vi "pulse_generator_data.vi"(4 "Record dP Data":refnum<vi>, 5 "queue in":refnum<queue>, 6 "Stop! Refnum":refnum<vi>, 7 "Recording Progressbar":refnum<vi>, 8 "Seesion Start Time":timestamp, 9 "Pulse Generator Chart Refnums":T3, 10 "Pulse Generator Offsets and Data Saving Controls Refnums":T2, 11 "Pulse Generator Measurement Refnums":T1) -> ()   [LabVIEW 2015]
uses:
  <vilib>/DAQmx/configure/timing.llb/DAQmx Timing (Sample Clock).vi
  <vilib>/DAQmx/read.llb/DAQmx Read (Analog 1D Wfm NChan NSamp).vi
  <vilib>/Waveform/WDTOps.llb/WDT Get Waveform Time Array DBL.vi
  pulse_generator_data_controls_refnums.ctl
  pulse_generator_data_refnums.ctl
  pulse_generator_data_charts_refnums.ctl
panel:
  out "size(s)":i32[](graph)
  out "Sampling Rate":refnum<vi>
  out "Recording Duration":refnum<vi>
  out "Camera Voltage Chart":refnum<vi>
  out "Abs Tank Pressure Chart":refnum<vi>
  out "Pitot dP Chart":refnum<vi>
  out "Pulse Generator to Test Section dP Chart":refnum<vi>
  out "W1-7 dP":refnum<vi>
  out "W1-4 dP":refnum<vi>
  out "Mass Flow Rate":refnum<vi>
  out "Liquid Sat Pressure":refnum<vi>
  out "Liquid Temperature":refnum<vi>
  out "Vapor Sat Pressure":refnum<vi>
  out "Vapor Temperature":refnum<vi>
  out "Pitot dP":refnum<vi>
  out "PG to TS dP":refnum<vi>
  out "Pitot Current":refnum<vi>
  out "PG Abs Pressure":refnum<vi>
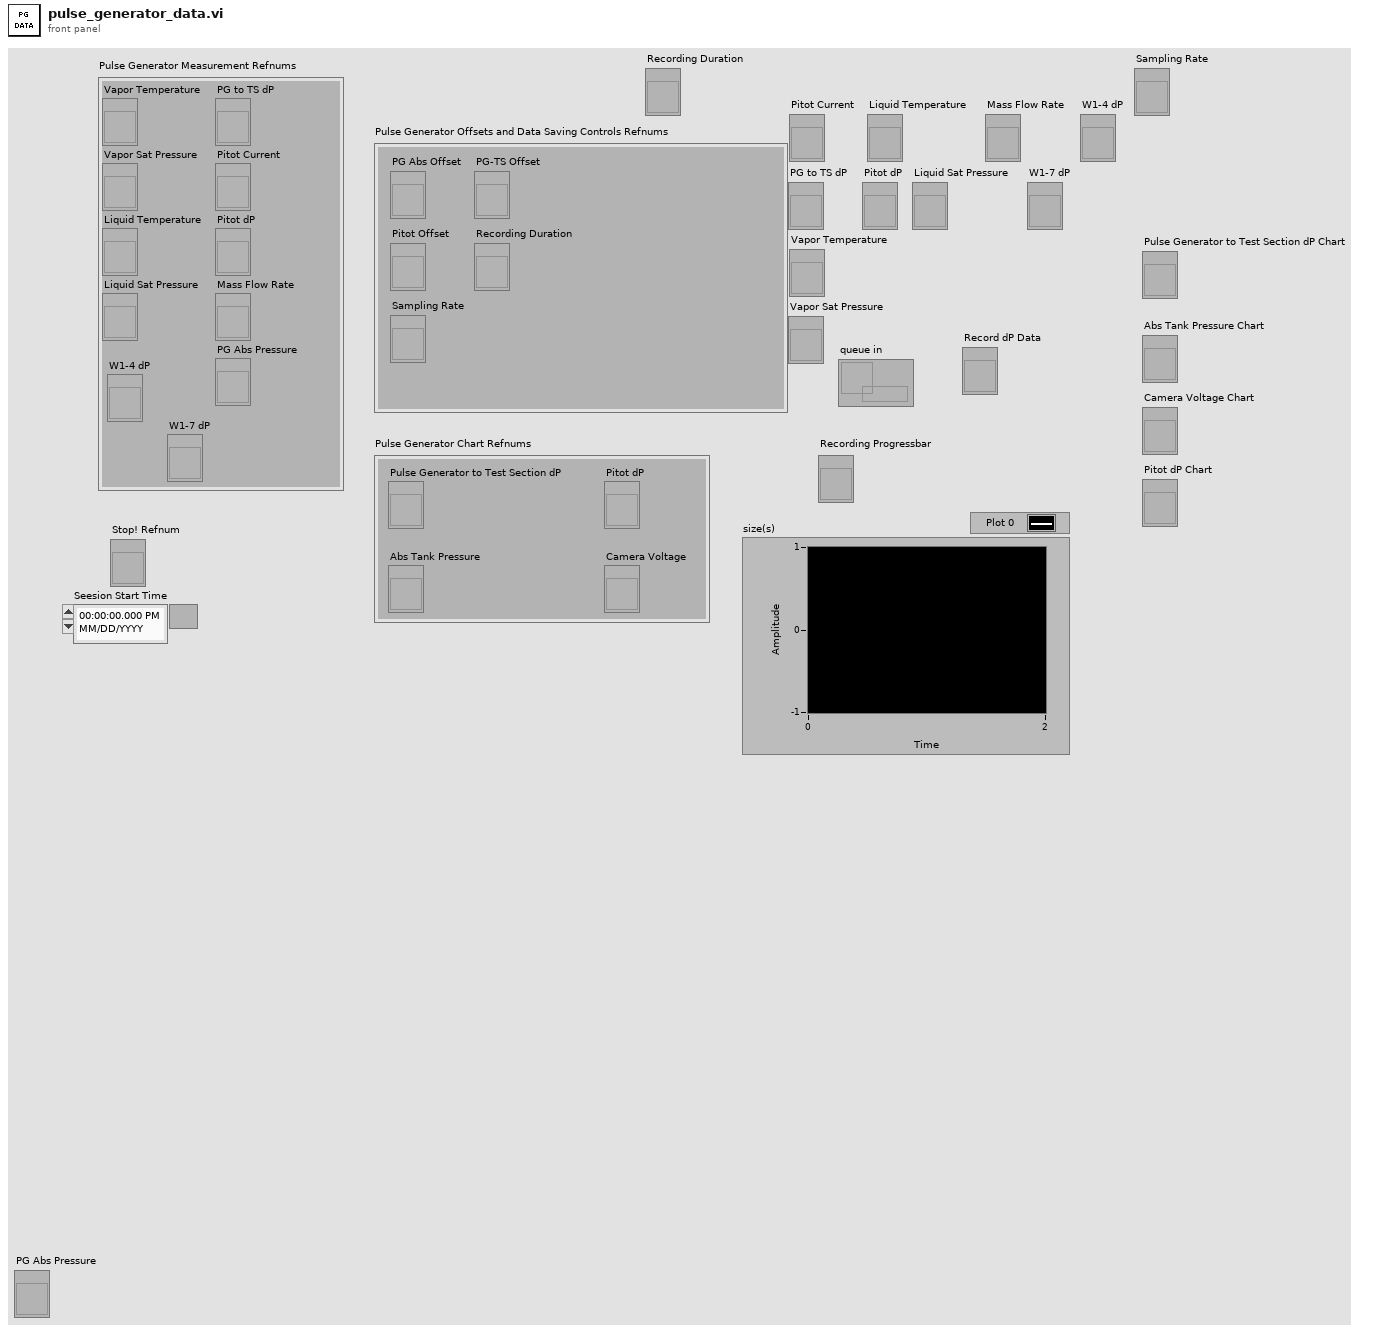
[diagram p1: front panel]
types:
  T1 = typedef "pulse_generator_data_refnums.ctl" = cluster{"Vapor Temperature":refnum<vi>, "Vapor Sat Pressure":refnum<vi>, "Liquid Temperature":refnum<vi>, "Liquid Sat Pressure":refnum<vi>, "PG to TS dP":refnum<vi>, "Pitot Current":refnum<vi>, "Pitot dP":refnum<vi>, "Mass Flow Rate":refnum<vi>, "PG Abs Pressure":refnum<vi>, "W1-4 dP":refnum<vi>, "W1-7 dP":refnum<vi>}
  T2 = typedef "pulse_generator_data_controls_refnums.ctl" = cluster{"PG Abs Offset":refnum<vi>, "Pitot Offset":refnum<vi>, "PG-TS Offset":refnum<vi>, "Recording Duration":refnum<vi>, "Sampling Rate":refnum<vi>}
  T3 = typedef "pulse_generator_data_charts_refnums.ctl" = cluster{"Pulse Generator to Test Section dP":refnum<vi>, "Pitot dP":refnum<vi>, "Abs Tank Pressure":refnum<vi>, "Camera Voltage":refnum<vi>}
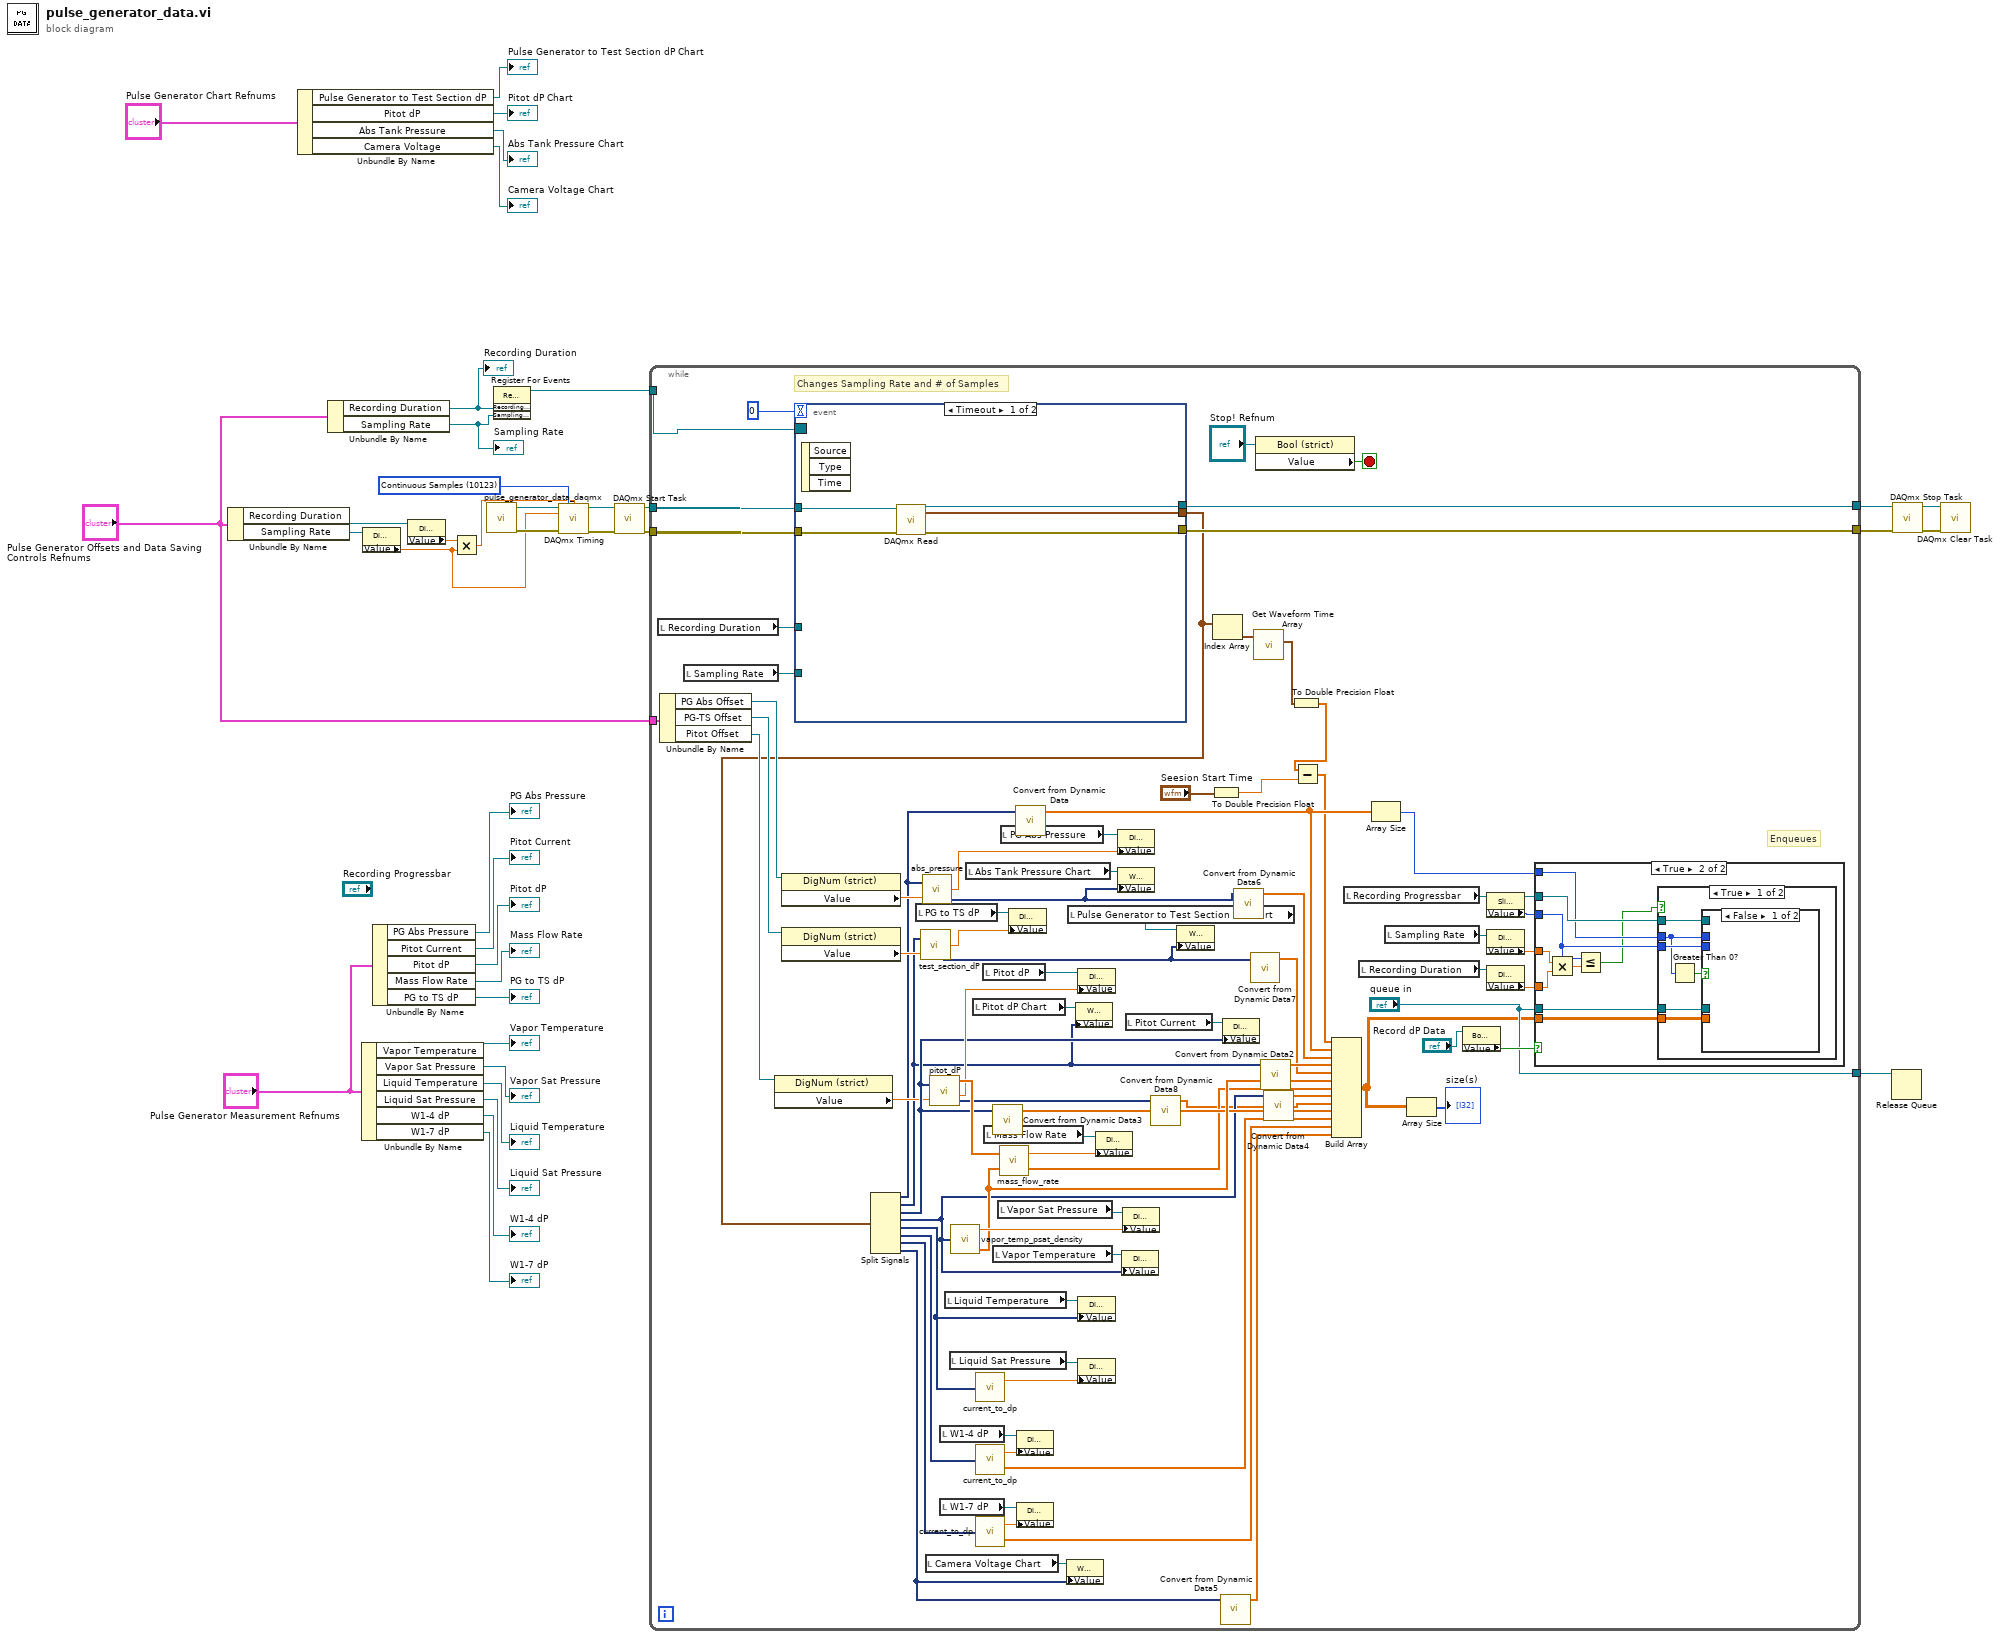
[diagram p0: block diagram]
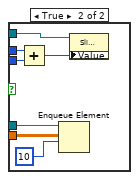
[diagram p3: hidden frame]
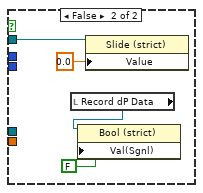
[diagram p4: hidden frame]
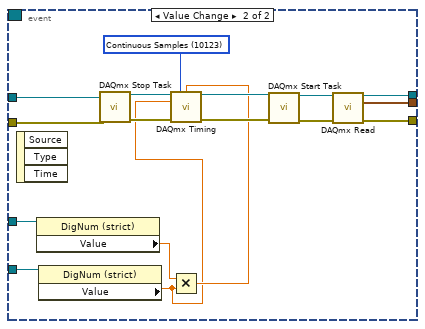
[diagram p5: hidden frame]
diagram:
  w34 = 10123 items=["Finite Samples"=10178, "Continuous Samples"=10123, "Hardware Timed Single Point"=12522] ("sample mode")
  n1 = Unbundle By Name("Pulse Generator Offsets and Data Saving Controls Refnums") -> ("Recording Duration"=w7:refnum<vi>, "Sampling Rate"=w2:refnum<vi>)
  n2 = Unbundle By Name("Pulse Generator Chart Refnums") -> ("Pulse Generator to Test Section dP"=→"Pulse Generator to Test Section dP Chart":refnum<vi>, "Pitot dP"=→"Pitot dP Chart":refnum<vi>, "Abs Tank Pressure"=→"Abs Tank Pressure Chart":refnum<vi>, "Camera Voltage"=→"Camera Voltage Chart":refnum<vi>)
  n3 = Unbundle By Name("Pulse Generator Offsets and Data Saving Controls Refnums") -> ("Recording Duration"=w5:refnum<vi>, "Sampling Rate"=w4:refnum<vi>)
  "Recording Duration" <- w5
  "Sampling Rate" <- w4
  n4 = Unbundle By Name("Pulse Generator Measurement Refnums") -> ("Vapor Temperature"=→"Vapor Temperature":refnum<vi>, "Vapor Sat Pressure"=→"Vapor Sat Pressure":refnum<vi>, "Liquid Temperature"=→"Liquid Temperature":refnum<vi>, "Liquid Sat Pressure"=→"Liquid Sat Pressure":refnum<vi>, "W1-4 dP"=→"W1-4 dP":refnum<vi>, "W1-7 dP"=→"W1-7 dP":refnum<vi>)
  n5 = property class="DigNum (strict)"(reference=w2) -> ("Value"=w3:dbl)  [unwired: 1 in, 2 out]
  n6 = Unbundle By Name("Pulse Generator Measurement Refnums") -> ("PG Abs Pressure"=→"PG Abs Pressure":refnum<vi>, "Pitot Current"=→"Pitot Current":refnum<vi>, "Pitot dP"=→"Pitot dP":refnum<vi>, "Mass Flow Rate"=→"Mass Flow Rate":refnum<vi>, "PG to TS dP"=→"PG to TS dP":refnum<vi>)
  n7 = property class="DigNum (strict)"(reference=w7) -> ("Value"=w10:dbl)  [unwired: 1 in, 2 out]
  n8 = Multiply(x=w10, y=w3) -> (x*y=w8:dbl)
  n9 = call "pulse_generator_data_daqmx.vi"() -> ("error out"=w11:errorcluster, "task out"=w35:refnum<k21>)  [unwired: 10 in]
  n10 = register-events(w5, w4) -> (reference out=w38:refnum<event-registration>)  [unwired: 2 in, 1 out]
  n11 = call-poly <vilib>:"DAQmx Timing.vi"("task/channels in"=w35, "sample mode"=w34, "samples per channel"=w8, "rate"=w3, "error in"=w11) -> ("task out"=w36:refnum<k21>, "error out"=w37:errorcluster)  [unwired: 9 in]
  n12 = call <vilib>:"DAQmx Start Task.vi"("task/channels in"=w36, "error in"=w37) -> ("task out"=w33:refnum<k21>, "error out"=w32:errorcluster)  [unwired: 12 in]
  n13 = while {
    tunnel: w38 -> [w122]
    tunnel: w33 -> [w121]
    tunnel: w32 -> [w120]
    tunnel: [w118] -> w31
    tunnel: [w117] -> w30
    tunnel: "Pulse Generator Offsets and Data Saving Controls Refnums" -> [w114]
    tunnel: ["queue in"] -> w9
    stop <- w115 stop-if-true
    # "Changes Sampling Rate and # of Samples"
    # "Enqueues"
    n14 = local read "Recording Duration"() -> (w67:refnum<vi>)
    n15 = Unbundle By Name(w114) -> ("PG Abs Offset"=w113:refnum<vi>, "PG-TS Offset"=w112:refnum<vi>, "Pitot Offset"=w111:refnum<vi>)
    n16 = local read "Sampling Rate"() -> (w66:refnum<vi>)
    n17 = property class="DigNum (strict)"(reference=w111) -> ("Value"=w57:dbl)  [unwired: 1 in, 2 out]
    n18 = property class="DigNum (strict)"(reference=w113) -> ("Value"=w110:dbl)  [unwired: 1 in, 2 out]
    n19 = property class="DigNum (strict)"(reference=w112) -> ("Value"=w62:dbl)  [unwired: 1 in, 2 out]
    n20 = event shown="[0] Timeout" {
      selector: w122 -> [_ _]
      dyn-events: _ -> [_ _]
      timeout: 0 -> [_ _]
      tunnel: w121 -> [w153 w170]
      tunnel: w120 -> [w152 w169]
      tunnel: [w149 w161] -> w118
      tunnel: [w150 w160] -> w117
      tunnel: [w151 w159] -> w45
      tunnel: w66 -> [_ w158]
      tunnel: w67 -> [_ w154]
      event Timeout {
        n21 = event-data() -> ()  [unwired: 1 in, 3 out]
        n22 = call-poly <vilib>:"DAQmx Read.vi"("task/channels in"=w153, "error in"=w152) -> ("task out"=w149:refnum<k21>, "data"=w151:waveform(dbl)[], "error out"=w150:errorcluster)  [unwired: 11 in]
      }
      event Value Change {
        w166 = 10123 items=["Finite Samples"=10178, "Continuous Samples"=10123, "Hardware Timed Single Point"=12522] ("sample mode")
        n23 = event-data() -> ()  [unwired: 1 in, 3 out]
        n24 = property class="DigNum (strict)"(reference=w154) -> ("Value"=w156:dbl)  [unwired: 1 in, 2 out]
        n25 = property class="DigNum (strict)"(reference=w158) -> ("Value"=w155:dbl)  [unwired: 1 in, 2 out]
        n26 = call <vilib>:"DAQmx Stop Task.vi"("task/channels in"=w170, "error in"=w169) -> ("task out"=w168:refnum<k21>, "error out"=w167:errorcluster)  [unwired: 12 in]
        n27 = Multiply(x=w156, y=w155) -> (x*y=w157:dbl)
        n28 = call-poly <vilib>:"DAQmx Timing.vi"("task/channels in"=w168, "sample mode"=w166, "samples per channel"=w157, "rate"=w155, "error in"=w167) -> ("task out"=w165:refnum<k21>, "error out"=w164:errorcluster)  [unwired: 9 in]
        n29 = call <vilib>:"DAQmx Start Task.vi"("task/channels in"=w165, "error in"=w164) -> ("task out"=w163:refnum<k21>, "error out"=w162:errorcluster)  [unwired: 12 in]
        n30 = call-poly <vilib>:"DAQmx Read.vi"("task/channels in"=w163, "error in"=w162) -> ("task out"=w161:refnum<k21>, "data"=w159:waveform(dbl)[], "error out"=w160:errorcluster)  [unwired: 11 in]
      }
    }
    n31 = Split Signals(w45) -> (w46:dynamicdata, w55:dynamicdata, w65:dynamicdata, w63:dynamicdata, w100:dynamicdata, w96:dynamicdata, w95:dynamicdata, w76:dynamicdata)  [unwired: 8 in]
    n32 = local read "PG to TS dP"() -> (w109:refnum<vi>)
    n33 = call "test_section_dP.vi"("dP Voltage"=w55, "Offset[Pa]"=w62) -> ("Adj dP"=w85:dbl, "Adj dP Array"=w49:dynamicdata)  [unwired: 1 out]
    n34 = call "abs_pressure.vi"("Input Voltage"=w46, "Offset[Pa]"=w110) -> ("Adj Absolute Pressure"=w86:dbl, "Adj Absolute Pressure Array"=w51:dynamicdata)  [unwired: 1 out]
    n35 = local read "Camera Voltage Chart"() -> (w87:refnum<vi>)
    n36 = call "pitot_dP.vi"("Pitot Current"=w65, "Pitot Offset [Pa]"=w57) -> ("dP H2O"=w105:dbl[], "Adj dP [Pa]"=w88:dbl, "Adj dP [Pa] Array"=w47:dynamicdata)  [unwired: 1 out]
    n37 = local read "W1-4 dP"() -> (w97:refnum<vi>)
    n38 = local read "W1-7 dP"() -> (w94:refnum<vi>)
    n39 = local read "Liquid Temperature"() -> (w101:refnum<vi>)
    n40 = local read "Liquid Sat Pressure"() -> (w103:refnum<vi>)
    n41 = call "vapor_temp_psat_density.vi"("Vapor Temp [C}"=w63) -> ("Psat Vapor"=w106:dbl, "Vapor Density Array"=w83:dbl[])  [unwired: 1 out]
    n42 = local read "Abs Tank Pressure Chart"() -> (w90:refnum<vi>)
    n43 = local read "Pitot dP Chart"() -> (w89:refnum<vi>)
    n44 = call "current_to_dp.vi"("Current [A]"=w100) -> ("dP [Pa]"=w102:dbl)  [unwired: 1 out]
    n45 = call "current_to_dp.vi"("Current [A]"=w96) -> ("dP [Pa]"=w98:dbl, "dP Array [Pa]"=w82:dbl[])
    n46 = call "current_to_dp.vi"("Current [A]"=w95) -> ("dP [Pa]"=w93:dbl, "dP Array [Pa]"=w64:dbl[])
    n47 = local read "Pitot dP"() -> (w107:refnum<vi>)
    n48 = local read "Mass Flow Rate"() -> (w104:refnum<vi>)
    n49 = call "Convert from Dynamic Data3"("Dynamic Data Type"=w65) -> ("Array"=w79:dbl[])  [unwired: 3 in]
    n50 = local read "Vapor Temperature"() -> (w99:refnum<vi>)
    n51 = local read "Vapor Sat Pressure"() -> (w92:refnum<vi>)
    n52 = call "mass_flow_rate.vi"("Density"=w83, "dP H2O"=w105) -> ("Mass Flow Rate [g/s] Array"=w61:dbl[], "Mass Flow Rate [g/s]"=w84:dbl)
    n53 = local read "PG Abs Pressure"() -> (w59:refnum<vi>)
    n54 = property class="DigNum (strict)"(reference=w109, "Value"=w85) -> ()  [unwired: 1 in, 2 out]
    n55 = call "Convert from Dynamic Data"("Dynamic Data Type"=w46) -> ("Array"=w75:dbl[])  [unwired: 3 in]
    n56 = property class="DigNum (strict)"(reference=w97, "Value"=w98) -> ()  [unwired: 1 in, 2 out]
    n57 = property class="DigNum (strict)"(reference=w94, "Value"=w93) -> ()  [unwired: 1 in, 2 out]
    n58 = property class="WFChart (strict)"(reference=w87, "Value"=w76) -> ()  [unwired: 1 in, 2 out]
    n59 = local read "Pulse Generator to Test Section dP Chart"() -> (w91:refnum<vi>)
    n60 = property class="WFChart (strict)"(reference=w89, "Value"=w55) -> ()  [unwired: 1 in, 2 out]
    n61 = property class="DigNum (strict)"(reference=w107, "Value"=w88) -> ()  [unwired: 1 in, 2 out]
    n62 = property class="DigNum (strict)"(reference=w101, "Value"=w100) -> ()  [unwired: 1 in, 2 out]
    n63 = property class="DigNum (strict)"(reference=w103, "Value"=w102) -> ()  [unwired: 1 in, 2 out]
    n64 = property class="DigNum (strict)"(reference=w104, "Value"=w84) -> ()  [unwired: 1 in, 2 out]
    n65 = property class="DigNum (strict)"(reference=w59, "Value"=w86) -> ()  [unwired: 1 in, 2 out]
    n66 = property class="WFChart (strict)"(reference=w90, "Value"=w51) -> ()  [unwired: 1 in, 2 out]
    n67 = property class="DigNum (strict)"(reference=w99, "Value"=w63) -> ()  [unwired: 1 in, 2 out]
    n68 = property class="DigNum (strict)"(reference=w92, "Value"=w106) -> ()  [unwired: 1 in, 2 out]
    n69 = local read "Pitot Current"() -> (w108:refnum<vi>)
    n70 = call "Convert from Dynamic Data8"("Dynamic Data Type"=w47) -> ("Array"=w48:dbl[])  [unwired: 3 in]
    n71 = property class="WFChart (strict)"(reference=w91, "Value"=w49) -> ()  [unwired: 1 in, 2 out]
    n72 = To Double Precision Float(number="Seesion Start Time") -> (double precision float=w40:dbl)
    n73 = Index Array(array=w45) -> (element=w44:waveform(dbl))  [unwired: 1 in]
    n74 = call "Convert from Dynamic Data5"("Dynamic Data Type"=w76) -> ("Array"=w77:dbl[])  [unwired: 3 in]
    n75 = property class="DigNum (strict)"(reference=w108, "Value"=w65) -> ()  [unwired: 1 in, 2 out]
    n76 = call "Convert from Dynamic Data6"("Dynamic Data Type"=w51) -> ("Array"=w52:dbl[])  [unwired: 3 in]
    n77 = call "Convert from Dynamic Data7"("Dynamic Data Type"=w49) -> ("Array"=w50:dbl[])  [unwired: 3 in]
    n78 = call-poly <vilib>:"Get Waveform Time Array.vi"("waveform in"=w44) -> ("X array"=w43:timestamp[])  [unwired: 9 in, 1 out]
    n79 = property class="Bool (strict)"(reference="Stop! Refnum") -> ("Value"=w115:bool)  [unwired: 1 in, 2 out]
    n80 = call "Convert from Dynamic Data2"("Dynamic Data Type"=w55) -> ("Array"=w80:dbl[])  [unwired: 3 in]
    n81 = call "Convert from Dynamic Data4"("Dynamic Data Type"=w63) -> ("Array"=w78:dbl[])  [unwired: 3 in]
    n82 = To Double Precision Float(number=w43) -> (double precision float=w42:dbl[])
    n83 = Subtract(x=w42, y=w40) -> (x-y=w39:dbl[])
    n84 = Build Array(w39, w75, w52, w80, w50, w83, w61, w78, w48, w79, w82, w64, w77) -> (w54:dbl[][])
    n85 = local read "Recording Progressbar"() -> (w69:refnum<vi>)
    n86 = local read "Recording Duration"() -> (w73:refnum<vi>)
    n87 = Array Size(array=w75) -> (size(s)=w58:i32)
    n88 = local read "Sampling Rate"() -> (w74:refnum<vi>)
    n89 = Array Size(array=w54) -> (size(s)=→"size(s)":i32[])
    n90 = property class="Bool (strict)"(reference="Record dP Data") -> ("Value"=w60:bool)  [unwired: 1 in, 2 out]
    n91 = property class="Slide (strict)"(reference=w69) -> (reference out=w68:refnum<vi>, "Value"=w70:u32)  [unwired: 1 in, 1 out]
    n92 = property class="DigNum (strict)"(reference=w74) -> ("Value"=w72:dbl)  [unwired: 1 in, 2 out]
    n93 = property class="DigNum (strict)"(reference=w73) -> ("Value"=w71:dbl)  [unwired: 1 in, 2 out]
    n94 = case shown="True" w60 {
      tunnel: "queue in" -> [_ w131]
      tunnel: w58 -> [_ w124]
      tunnel: w72 -> [_ w130]
      tunnel: w71 -> [_ w129]
      tunnel: w70 -> [_ w127]
      tunnel: w68 -> [_ w126]
      tunnel: w54 -> [_ w125]
      frame False {
      }
      frame True {
        n95 = Multiply(x=w130, y=w129) -> (x*y=w128:dbl)
        n96 = Less Or Equal?(x=w127, y=w128) -> (x <= y?=w123:bool)
        n97 = case shown="True" w123 {
          tunnel: w131 -> [w137 _]
          tunnel: w126 -> [w136 w148]
          tunnel: w127 -> [w135 _]
          tunnel: w124 -> [w132 _]
          tunnel: w125 -> [w134 _]
          frame True {
            n98 = Greater Than 0?(x=w132) -> (x > 0?=w133:bool)
            n99 = case shown="False" w133 {
              tunnel: w137 -> [_ w143]
              tunnel: w136 -> [_ w142]
              tunnel: w135 -> [_ w140]
              tunnel: w132 -> [_ w139]
              tunnel: w134 -> [_ w138]
              frame False {
              }
              frame True {
                n100 = Add(x=w139, y=w140) -> (x+y=w141:u32)
                n101 = Enqueue Element(queue=w143, element=w138, timeout in ms (-1)=10) -> ()  [unwired: 1 in, 3 out]
                n102 = property class="Slide (strict)"(reference=w142, "Value"=w141) -> ()  [unwired: 1 in, 2 out]
              }
            }
          }
          frame False {
            n103 = local read "Record dP Data"() -> (w145:refnum<vi>)
            n104 = property class="Bool (strict)"(reference=w145, "Val(Sgnl)"=FALSE ("Value (Signaling)")) -> ()  [unwired: 1 in, 2 out]
            n105 = property class="Slide (strict)"(reference=w148, "Value"=0.0) -> ()  [unwired: 1 in, 2 out]
          }
        }
      }
    }
  }
  n106 = Release Queue(queue=w9) -> ()  [unwired: 2 in, 3 out]
  n107 = call <vilib>:"DAQmx Stop Task.vi"("task/channels in"=w31, "error in"=w30) -> ("task out"=w29:refnum<k21>, "error out"=w28:errorcluster)  [unwired: 12 in]
  n108 = call <vilib>:"DAQmx Clear Task.vi"("task in"=w29, "error in"=w28) -> ()  [unwired: 13 in, 1 out]
